vi "Read configuration.vi"(7 "force loading?":bool=TRUE, 8 "error in (no error)":errorcluster, 11 "StageSPIM in":refnum<class "StageSPIM.lvclass">) -> (0 "error out":errorcluster, 3 "StageSPIM out":refnum<class "StageSPIM.lvclass">)   [LabVIEW 2012, in "StageSPIM.lvclass"]
doc: "Reads the XML-based configuration file and populates the configuration cluster accordingly. Configuration file name is <component ID>.xml."
uses:
  StageSPIM.lvclass
  <vilib>/Distrio/Murmex/Murmex/Murmex.lvclass
  StageSPIM.lvclass/StageSPIM.ctl
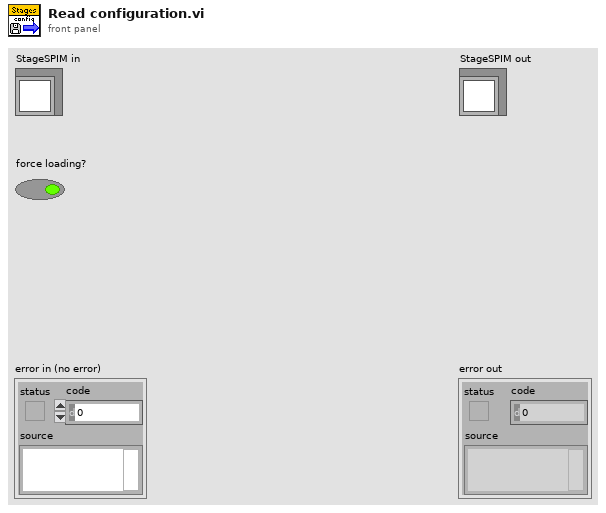
[diagram p1: front panel]
types:
  T1 = typedef "StageSPIM.lvclass/configuration_cluster.ctl" = cluster{"Port":T2, "Baudrate":T3, "Update frequency":dbl[unit], "S/N Master controller":string, "Interface":T4, "soft min limit":dbl[], "soft max limit":dbl[], "startup speedX":dbl[unit], "startup speedY":dbl[unit], "startup speedZ":dbl[unit], "startup speedFocus":dbl[unit]}
  T2 = typedef "StageSPIM.lvclass/port_control.ctl" = i32
  T3 = typedef "StageSPIM.lvclass/baud_rate_control.ctl" = u16
  T4 = typedef "StageSPIM.lvclass/connection_type.ctl" = enum16{"RS232", "RS232 DaisyChain", "USB", "USB_DaisyChain"}
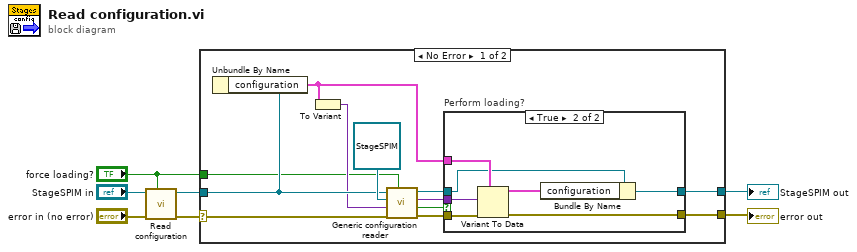
[diagram p0: block diagram]
diagram:
  n1 = call-parent "Read configuration.vi"("force loading?"="force loading?", "error in (no error)"="error in (no error)", "Murmex in"="StageSPIM in") -> ("error out"=w5:errorcluster, "Murmex out"=w4:refnum<class "StageSPIM.lvclass">)  [unwired: 7 in]
  n2 = case shown="No Error" w5 {
    selector: w5 -> [w17 w29]
    tunnel: w4 -> [w18 w30]
    tunnel: "force loading?" -> [w15 _]
    tunnel: [w9 w30] -> w2
    tunnel: [w8 w29] -> w1
    frame No Error {
      n3 = Unbundle By Name(w18) -> ("configuration"=w13:T1)
      n4 = To Variant(anything=w13) -> (Variant=w16:variant)
      n5 = call <vilib>:"Generic configuration reader.vi"("force loading?"=w15, "error in (no error)"=w17, "configuration cluster variant"=w16, "inheritance level"=refnum<class "StageSPIM.lvclass"> refnum ("StageSPIM.lvclass"), "Murmex in"=w18) -> ("error out"=w14:errorcluster, "loaded?"=w11:bool, "configuration data (variant)"=w10:variant, "Murmex out"=w12:refnum<class "StageSPIM.lvclass">)  [unwired: 3 in]
      n6 = case "Perform loading?" shown="True" w11 {
        tunnel: w13 -> [_ w28]
        tunnel: [w21 w26] -> w8
        tunnel: [w20 w25] -> w9
        tunnel: w14 -> [w21 w22]
        tunnel: w12 -> [w20 w24]
        tunnel: w10 -> [_ w23]
        frame False {
        }
        frame True {
          n7 = Variant To Data(error in=w22, type=w28, Variant=w23) -> (data=w27:T1, error out=w26:errorcluster)
          n8 = Bundle By Name(cluster=w24, "configuration"=w27) -> (w25:refnum<class "StageSPIM.lvclass">)
        }
      }
    }
    frame Error {
    }
  }
  "error out" <- w1
  "StageSPIM out" <- w2
